vi "Export ALL Settings (ZIP File).vi"(0 "reference in":refnum<class "Generic Utilities.lvclass">, 5 "error in (no error)":errorcluster) -> (14 "reference out":refnum<class "Generic Utilities.lvclass">, 19 "error out":errorcluster)   [LabVIEW 2020, in "Generic Utilities.lvclass"]
uses:
  Generic Utilities.lvclass
  <vilib>/Utility/sysdir.llb/System Directory Type.ctl
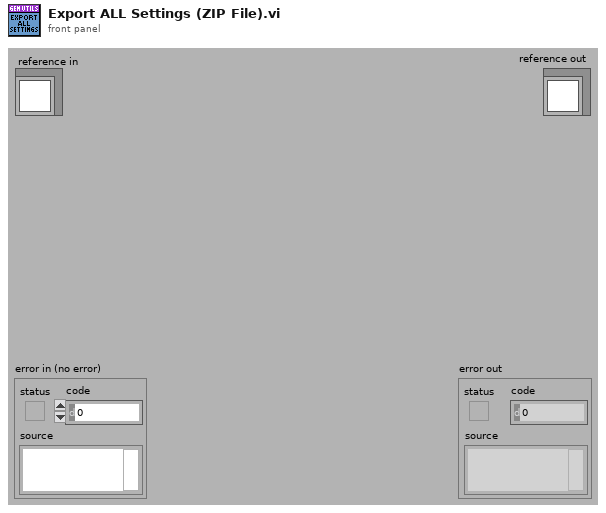
[diagram p1: front panel]
types:
  T1 = typedef "System Directory Type.ctl" = i32
  T2 = typedef "Generic Utilities.lvclass/ObjectAttributes.ctl" = cluster{"GUI Parameters":T3, "State Machine Control":cluster{"Timeout":i32, "State Queue":string[], "State History":string[], "State History Length":i32}, "Logging File Path":path, "OBJ not a refnum?":bool, "Timer Start":timestamp, "FP Refnums":T4}
  T3 = typedef "Generic Utilities.lvclass/GUI Parameters.ctl" = cluster{"Application Name":string, "GUI VI Ref":refnum<vi>, "Close Panel?":bool, "Message Window ref":refnum<vi>, "Version #":string}
  T4 = typedef "Generic Utilities.lvclass/FP Refnums.ctl" = cluster{"Panel refnum":refnum<vi>, "Control Labels":string[], "Refnums":refnum<vi>[]}
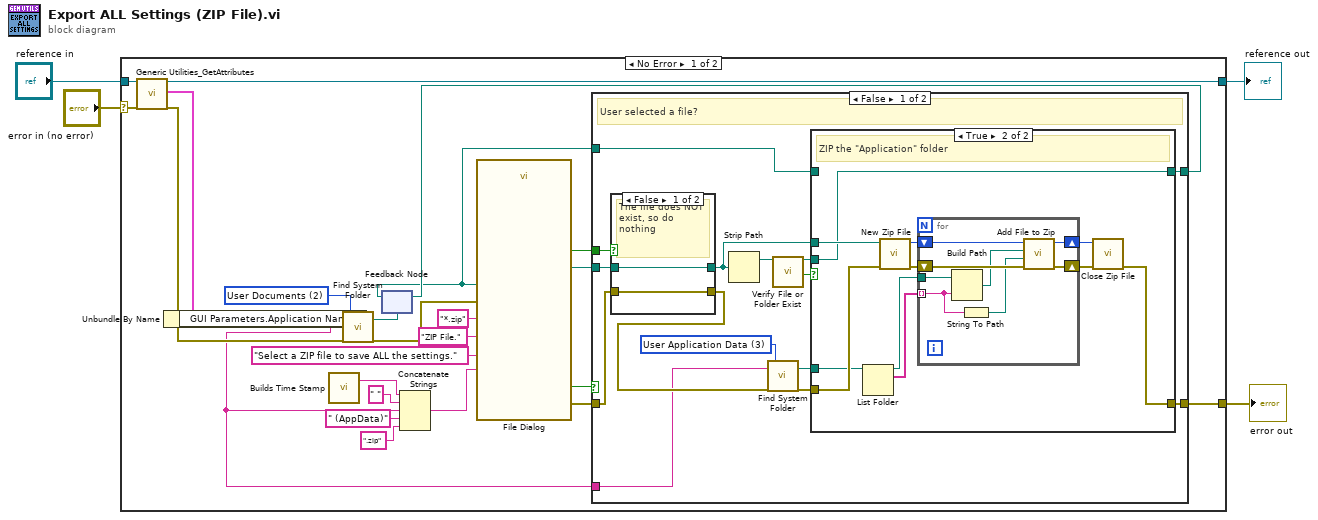
[diagram p0: block diagram]
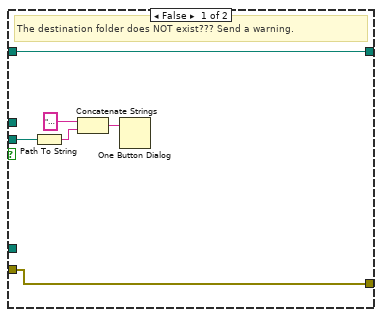
[diagram p2: hidden frame]
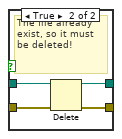
[diagram p3: hidden frame]
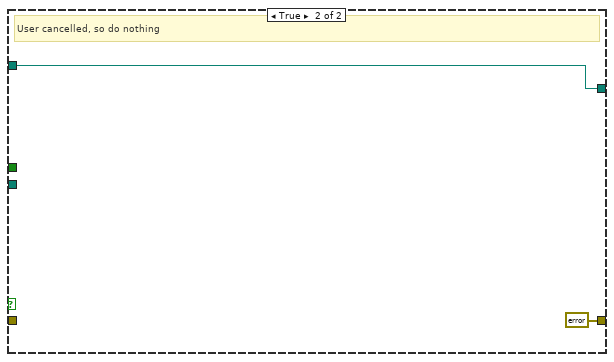
[diagram p4: hidden frame]
diagram:
  n1 = case shown="No Error" "error in (no error)" {
    selector: "error in (no error)" -> [w28 w78]
    tunnel: [w9 w78] -> w3
    tunnel: [w27 w77] -> w1
    tunnel: "reference in" -> [w25 w77]
    frame No Error {
      w23 = T1 2 items=["User Home"=0, "User Desktop"=1, "User Documents"=2, "User Application Data"=3, "User Preferences"=4, "User Temporary"=5, "Public Documents"=6, "Public Application Data"=7, "Public Preferences"=8, "Public Cache"=13, "System Core Libraries"=9, "System Installed Libraries"=10, "Application Files"=11, "Boot Volume Root"=12] ("system directory type")
      n2 = call "Generic Utilities_GetAttributes.vi"("reference in"=w25, "error in (no error)"=w28) -> ("reference out"=w27:refnum<class "Generic Utilities.lvclass">, "attributes"=w26:T2, "error out"=w24:errorcluster)  [unwired: 14 in, 1 out]
      n3 = Unbundle By Name(w26) -> ("GUI Parameters.Application Name"=w10:string)
      n4 = call "Builds Time Stamp.vi"() -> ("TimeStamp"=w16:string)  [unwired: 19 in]
      n5 = call "Find System Folder.vi"("Application Name"=w10, "error in (no error)"=w24, "system directory type"=w23) -> ("System Folder"=w22:path, "error out"=w20:errorcluster)  [unwired: 15 in]
      n6 = feedback #1(w22) -> (w7:path)
      n7 = Concatenate Strings(w16, " " ("string"), w10, " (AppData)" ("string"), ".zip" ("string")) -> (w14:string)
      n8 = call "File Dialog"("start path"=w7, "prompt"="Select a ZIP file to save ALL the settings.", "default name"=w14, "error in"=w20, "pattern (all files)"="*.zip" ("pattern label"), "pattern label"="ZIP File.") -> ("selected path"=w21:path, "exists"=w12:bool, "cancelled"=w13:bool, "error out"=w11:errorcluster)  [unwired: 6 in]
      n9 = case shown="False" w13 {
        tunnel: w21 -> [w41 _]
        tunnel: w12 -> [w42 _]
        tunnel: w11 -> [w40 _]
        tunnel: w10 -> [w35 _]
        tunnel: [w31 errorcluster {"status"=FALSE, "code"=0, "source"=""} ("error out")] -> w9
        tunnel: [w30 w75] -> w8
        tunnel: w7 -> [w29 w75]
        frame False {
          w37 = T1 3 items=["User Home"=0, "User Desktop"=1, "User Documents"=2, "User Application Data"=3, "User Preferences"=4, "User Temporary"=5, "Public Documents"=6, "Public Application Data"=7, "Public Preferences"=8, "Public Cache"=13, "System Core Libraries"=9, "System Installed Libraries"=10, "Application Files"=11, "Boot Volume Root"=12] ("system directory type")
          # "User selected a file?"
          n10 = case shown="False" w42 {
            tunnel: w41 -> [w70 w74]
            tunnel: w40 -> [w69 w73]
            tunnel: [w70 w72] -> w34
            tunnel: [w69 w71] -> w36
            frame False {
              # "The file does NOT exist, so do nothing"
            }
            frame True {
              # "The file already exist, so it must be deleted!"
              n11 = Delete(path (use dialog)=w74, error in=w73) -> (deleted path=w72:path, error out=w71:errorcluster)  [unwired: 3 in, 1 out]
            }
          }
          n12 = Strip Path(path=w34) -> (stripped path=w43:path)  [unwired: 1 out]
          n13 = call "Find System Folder.vi"("Application Name"=w35, "error in (no error)"=w36, "system directory type"=w37) -> ("System Folder"=w32:path, "error out"=w33:errorcluster)  [unwired: 15 in]
          n14 = call "Verify File or Folder Exist.vi"("path"=w43) -> ("dup path"=w38:path, "file or folder exists?"=w39:bool)  [unwired: 16 in, 1 out]
          n15 = case shown="True" w39 {
            tunnel: w38 -> [w49 w50]
            tunnel: w34 -> [_ w60]
            tunnel: w33 -> [w45 w59]
            tunnel: w32 -> [_ w56]
            tunnel: [w45 w51] -> w31
            tunnel: [w44 w50] -> w30
            tunnel: w29 -> [w44 _]
            frame False {
              # "The destination folder does NOT exist??? Send a warning."
              n16 = Path To String(path=w49) -> (string=w47:string)
              n17 = Concatenate Strings("The following path does NOT exist?  Cannot export the application settings to that location?\n", w47) -> (w46:string)
              n18 = One Button Dialog(message=w46) -> ()  [unwired: 1 in, 1 out]
            }
            frame True {
              # "ZIP the \"Application\" folder"
              n19 = List Folder(path=w56) -> (path out=w54:path, filenames=w53:string[])  [unwired: 3 in, 2 out]
              n20 = call <vilib>:"New Zip File.vi"("error in (no error)"=w59, "target"=w60) -> ("error out"=w55:errorcluster, "zip file out"=w58:i64)  [unwired: 3 in, 1 out]
              n21 = for {
                shift-right: [w67] -> w57
                shift-left: w58 -> [w68]
                shift-right: [w66] -> w52
                shift-left: w55 -> [w65]
                tunnel: w54 -> [w64]
                tunnel: w53 -> [w62] mode=indexing
                n22 = Build Path(base path=w64, name or relative path=w62) -> (appended path=w63:path)
                n23 = String To Path(string=w62) -> (path=w61:path)
                n24 = call <vilib>:"Add File to Zip.vi"("error in (no error)"=w65, "destination path in zip"=w61, "source file path"=w63, "zip file in"=w68) -> ("error out"=w66:errorcluster, "zip file out"=w67:i64)  [unwired: 6 in]
              }
              n25 = call <vilib>:"Close Zip File.vi"("error in (no error)"=w52, "zip file in"=w57) -> ("error out"=w51:errorcluster)  [unwired: 5 in]
            }
          }
        }
        frame True {
          # "User cancelled, so do nothing"
        }
      }
      n26 = feedback-in #1(w8) -> ()
    }
    frame Error {
    }
  }
  "error out" <- w3
  "reference out" <- w1
